vi "堆栈（DBL）.vi"(6 "堆栈长度":i32=256, 8 "error in (no error)":errorcluster caption="错误输入（无错误）", 9 "堆栈操作":T1, 11 "入栈元素(DBL)":dbl) -> (0 "error out":errorcluster caption="错误输出", 1 "已用堆栈长度":i32, 2 "预览":dbl[](array[numeric]), 3 "出栈元素":dbl, 4 "堆栈空":bool, 5 "堆栈满":bool)   [LabVIEW 2012, in "Array Stack.lvlib"]
uses:
  Array Stack.lvlib
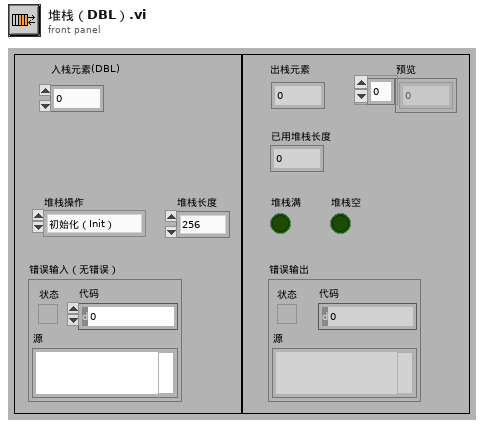
[diagram p1: front panel]
types:
  T1 = typedef "Array Stack.lvlib/堆栈操作.ctl" = enum16{"初始化（Init）", "进栈（Push）", "出栈（Pop）", "状态（Status)", "释放"}
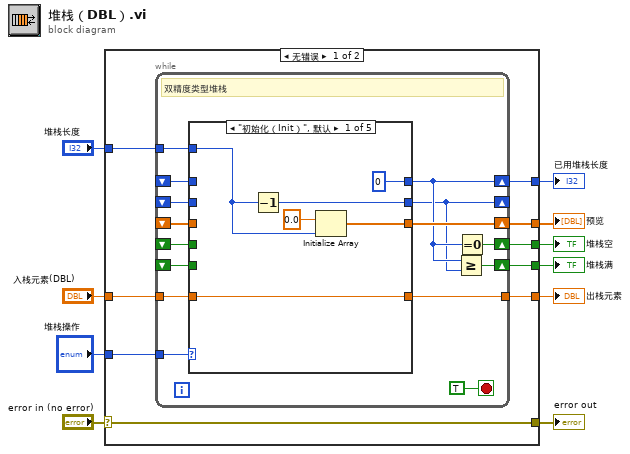
[diagram p0: block diagram]
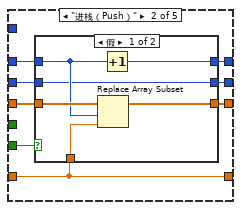
[diagram p2: hidden frame]
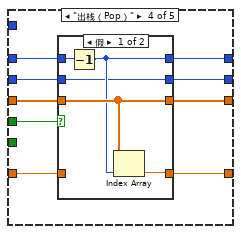
[diagram p5: hidden frame]
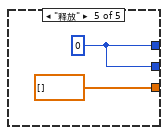
[diagram p7: hidden frame]
diagram:
  n1 = case shown="无错误" "error in (no error)" {
    selector: "error in (no error)" -> [w19 w81]
    tunnel: [w19 w81] -> w9
    tunnel: "堆栈操作" -> [w18 _]
    tunnel: "入栈元素(DBL)" -> [w17 _]
    tunnel: [w16 _] -> w6
    tunnel: [w12 _] -> w5
    tunnel: "堆栈长度" -> [w13 _]
    tunnel: [w15 _] -> w2
    tunnel: [w14 _] -> w3
    tunnel: [w11 _] -> w1
    frame No Error {
      n2 = while "While循环" {
        tunnel: w18 -> [w34]
        tunnel: w17 -> [w33]
        tunnel: [w32] -> w16
        tunnel: w13 -> [w30]
        shift-right: [w31] -> w11
        shift-left: _ -> [w27]
        shift-right: [w20] -> _
        shift-left: _ -> [w21]
        shift-right: [w24] -> w12
        shift-left: _ -> [w22]
        shift-right: [w26] -> w15
        shift-left: _ -> [w28]
        shift-right: [w25] -> w14
        shift-left: _ -> [w23]
        stop <- TRUE stop-if-true
        # "双精度类型堆栈"
        n3 = case shown="\"初始化（Init）\", 默认" w34 {
          tunnel: w33 -> [w40 w48 _ w63 _]
          tunnel: [w40 w48 _ w65 _] -> w32
          tunnel: [0 ("堆栈长度") w46 w60 w67 w79] -> w24
          tunnel: [w38 w44 w58 w64 dbl[] []] -> w31
          tunnel: w30 -> [w35 _ _ _ _]
          tunnel: w22 -> [_ w47 w60 w68 _]
          tunnel: w21 -> [_ w42 w59 w62 _]
          tunnel: w28 -> [_ w43 _ _ _]
          tunnel: w27 -> [_ w45 w58 w66 _]
          tunnel: w23 -> [_ _ _ w69 _]
          tunnel: [w36 w41 w59 w61 w79] -> w20
          frame "初始化（Init）", Default {
            n4 = Decrement(x=w35) -> (x-1=w36:i32)
            n5 = Initialize Array(0.0 ("入栈元素"), w35) -> (w38:dbl[])
          }
          frame "进栈（Push）" {
            n6 = case shown="假" w43 {
              tunnel: w48 -> [w53 _]
              tunnel: w47 -> [w50 w57]
              tunnel: [w54 w57] -> w46
              tunnel: w45 -> [w51 w56]
              tunnel: [w52 w56] -> w44
              tunnel: w42 -> [w49 w55]
              tunnel: [w49 w55] -> w41
              frame False {
                n7 = Replace Array Subset(array=w51, new element=w53, index=w50) -> (w52:dbl[])
                n8 = Increment(x=w50) -> (x+1=w54:i32)
              }
              frame True {
              }
            }
          }
          frame "状态（Status)" {
          }
          frame "出栈（Pop）" {
            n9 = case shown="假" w69 {
              tunnel: w68 -> [w72 w76]
              tunnel: [w71 w76] -> w67
              tunnel: w66 -> [w73 w78]
              tunnel: [w74 w77] -> w65
              tunnel: [w73 w78] -> w64
              tunnel: w63 -> [_ w77]
              tunnel: w62 -> [w70 w75]
              tunnel: [w70 w75] -> w61
              frame False {
                n10 = Decrement(x=w72) -> (x-1=w71:i32)
                n11 = Index Array(array=w73, index=w71) -> (element=w74:dbl)
              }
              frame True {
              }
            }
          }
          frame "释放" {
            w79 = 0 ("堆栈长度")
          }
        }
        n12 = Greater Or Equal?(x=w24, y=w20) -> (x >= y?=w26:bool)
        n13 = Equal To 0?(x=w24) -> (x = 0?=w25:bool)
      }
    }
    frame Error {
    }
  }
  "error out" <- w9
  "出栈元素" <- w6
  "已用堆栈长度" <- w5
  "堆栈满" <- w2
  "堆栈空" <- w3
  "预览" <- w1
